vi "Self Test All.vi"(8 "error in":errorcluster) -> (0 "error out":errorcluster, 2 "Step.Result":string, 3 "OK?":bool)   [LabVIEW 2023, in "LTT_TeststandSteptypes.lvlib"]
uses:
  LTT_TeststandSteptypes.lvlib
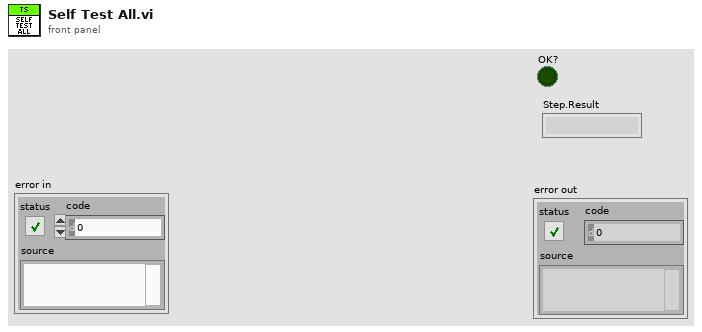
[diagram p1: front panel]
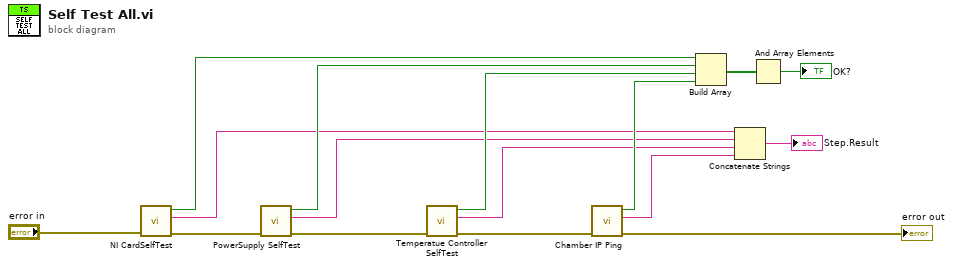
[diagram p0: block diagram]
diagram:
  n1 = call "NI CardSelfTest.vi"("error in"="error in") -> ("error out"=w16:errorcluster, "Report Text"=w6:string, "OK"=w10:bool)  [unwired: 8 in]
  n2 = call "PowerSupply SelfTest.vi"("error in"=w16) -> ("error out"=w15:errorcluster, "Report Text"=w5:string, "OK"=w11:bool)  [unwired: 8 in]
  n3 = call "Temperatue Controller SelfTest.vi"("error in"=w15) -> ("error out"=w14:errorcluster, "Report Text"=w4:string, "OK"=w12:bool)  [unwired: 8 in]
  n4 = call "Chamber IP Ping.vi"("error in (no error)"=w14) -> ("error out"=→"error out":errorcluster, "Report Text"=w3:string, "Chamber IP Ping?"=w13:bool)  [unwired: 8 in]
  n5 = Build Array(w10, w11, w12, w13) -> (w8:bool[])
  n6 = Concatenate Strings(w6, w5, w4, w3) -> (→"Step.Result":string)
  n7 = And Array Elements(Boolean array=w8) -> (logical AND=→"OK?":bool)
